vi "draw.vi"(0 "reference":refnum<class "SystemNode.lvclass">, 1 "graphics":refnum<class "Graphics.lvclass">, 5 "error in (no error)":errorcluster) -> (14 "reference out":refnum<class "SystemNode.lvclass">, 19 "error out":errorcluster)   [LabVIEW 2016, in "SystemNode.lvclass"]
doc: "public void draw(Graphics2D g2)"
uses:
  <resource>/Framework/Providers/Open_GDS/UML/SystemNode_class/SystemNode.lvclass
  C:/Program Files (x86)/National Instruments/LabVIEW 2016/resource/Framework/Providers/Open_GDS/UML/RectangularNode_class/RectangularNode.lvclass
  <resource>/Framework/Providers/Open_GDS/UML/Graphics_class/Graphics.lvclass
  <resource>/Framework/Providers/Open_GDS/UML/MultiLineString_class/MultiLineString.lvclass
  <resource>/Framework/Providers/Open_GDS/UML/RectangularNode_class/RectangularNode.lvclass
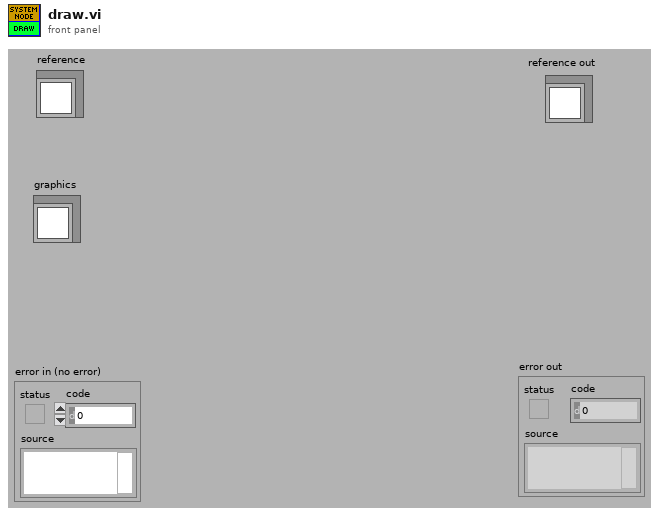
[diagram p1: front panel]
types:
  T1 = typedef "SystemNode.lvclass/ObjectAttributes.ctl" = cluster{"contents":refnum<class "MultiLineString.lvclass">, "DEFAULT_WIDTH":i32, "DEFAULT_HEIGHT":i32, "NAME_GAP":i32, "XGAP":i32, "YGAP":i32}
  T2 = typedef "RectangularNode.lvclass/ObjectAttributes.ctl" = cluster{"bounds":T3}
  T3 = typedef "Rectangle Rectangle2D.ctl" = cluster{"x":dbl, "y":dbl, "width":dbl, "height":dbl}
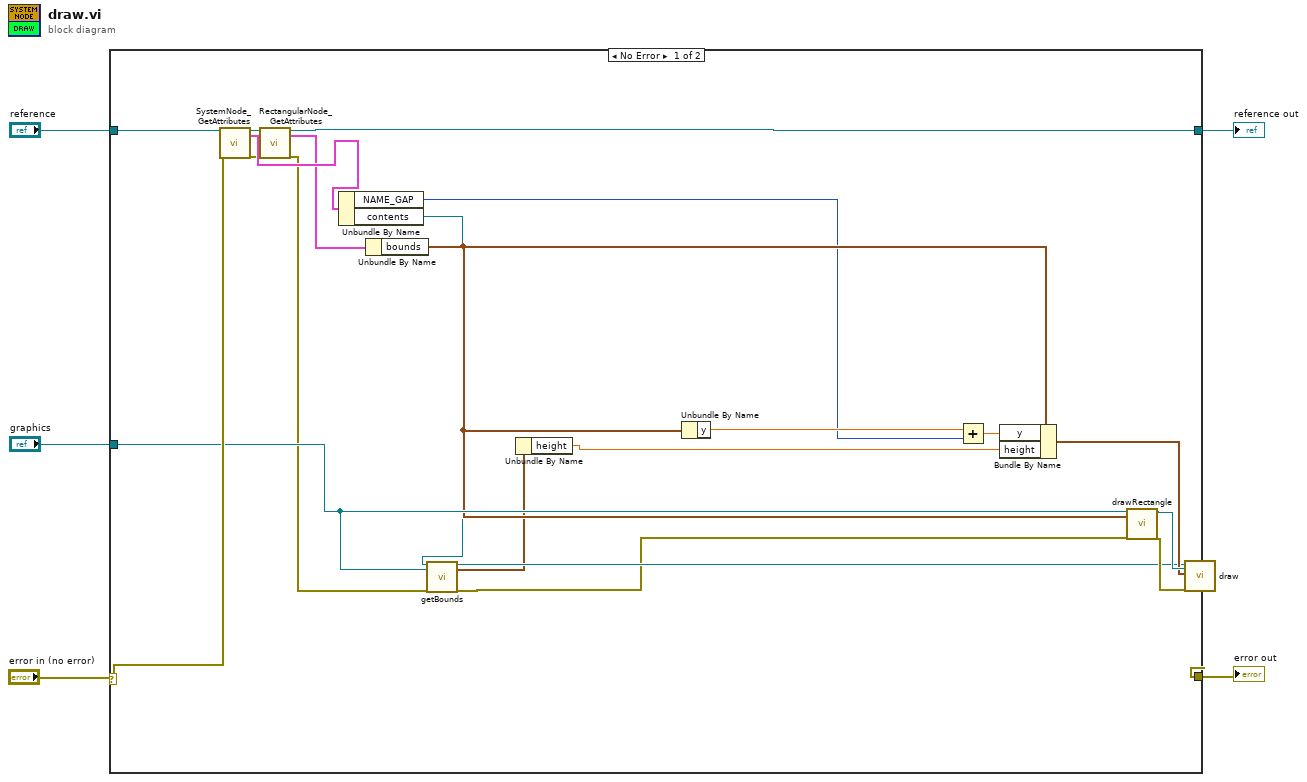
[diagram p0: block diagram]
diagram:
  n1 = case shown="No Error" "error in (no error)" {
    selector: "error in (no error)" -> [w25 w28]
    tunnel: "reference" -> [w27 w29]
    tunnel: [w26 w28] -> w4
    tunnel: [w7 w29] -> w3
    tunnel: "graphics" -> [w24 _]
    frame No Error {
      n2 = call <resource>:"SystemNode_GetAttributes.vi"("reference in"=w27, "error in (no error)"=w25) -> ("reference out"=w10:refnum<class "SystemNode.lvclass">, "Data"=w11:T1, "error out"=w9:errorcluster)  [unwired: 1 in, 14 out]
      n3 = call <resource>:"RectangularNode_GetAttributes.vi"("reference in"=w10, "error in (no error)"=w9) -> ("reference out"=w7:refnum<class "SystemNode.lvclass">, "Data"=w6:T2, "error out"=w8:errorcluster)  [unwired: 14 in, 1 out]
      n4 = Unbundle By Name(w11) -> ("NAME_GAP"=w13:i32, "contents"=w17:refnum<class "MultiLineString.lvclass">)
      n5 = Unbundle By Name(w6) -> ("bounds"=w18:T3)
      n6 = call-dynamic "getBounds.vi"("reference"=w17, "graphics"=w24, "error in (no error)"=w8) -> ("reference out"=w16:refnum<class "MultiLineString.lvclass">, "bounds"=w14:T3, "error out"=w15:errorcluster)  [unwired: 14 in]
      n7 = Unbundle By Name(w14) -> ("height"=w12:dbl)
      n8 = Unbundle By Name(w18) -> ("y"=w20:dbl)
      n9 = Add(x=w20, y=w13) -> (x+y=w23:dbl)
      n10 = Bundle By Name(cluster=w18, "y"=w23, "height"=w12) -> (w19:T3)
      n11 = call <resource>:"drawRectangle.vi"("reference"=w24, "rectangle"=w18, "error in (no error)"=w15) -> ("reference out"=w21:refnum<class "Graphics.lvclass">, "error out"=w22:errorcluster)  [unwired: 4 in, 11 out]
      n12 = call-dynamic "draw.vi"("reference"=w16, "graphics"=w21, "bounds"=w19, "error in (no error)"=w22) -> ("error out"=w26:errorcluster)  [unwired: 14 in, 1 out]
    }
    frame Error {
    }
  }
  "reference out" <- w3
  "error out" <- w4
